vi "set x And y As Point (I32).vi"(10 "Point":T1, 11 "Vector 2D in":refnum<class "Vector 2D.lvclass">) -> (3 "Vector 2D out":refnum<class "Vector 2D.lvclass">)   [LabVIEW 2021, in "Vector 2D.lvclass"]
uses:
  Vector 2D.lvclass
  Vector 2D.lvclass/Vector 2D.ctl
  LabSDL2/Source/Libraries/SDL2 Utility/Point (I32).ctl
  LabSDL2/Source/Libraries/SDL2 Utility/SDL2 Utility.lvlib
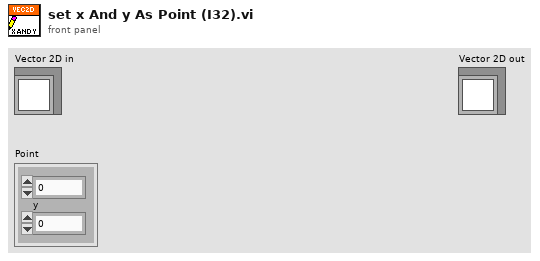
[diagram p1: front panel]
types:
  T1 = typedef "SDL2 Utility.lvlib/Point (I32).ctl" = cluster{"x":i32, "y":i32}
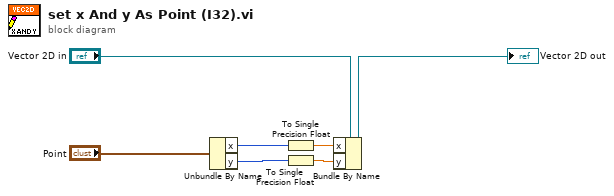
[diagram p0: block diagram]
diagram:
  n1 = Unbundle By Name("Point") -> ("x"=w4:i32, "y"=w2:i32)
  n2 = To Single Precision Float(number=w4) -> (single precision float=w3:sgl)
  n3 = To Single Precision Float(number=w2) -> (single precision float=w1:sgl)
  n4 = Bundle By Name(cluster="Vector 2D in", "x"=w3, "y"=w1) -> (→"Vector 2D out":refnum<class "Vector 2D.lvclass">)
